vi "PulseSplitBools.vi"(1 "Pulse input":T2) -> (0 "output cluster":T1)   [LabVIEW 2017]
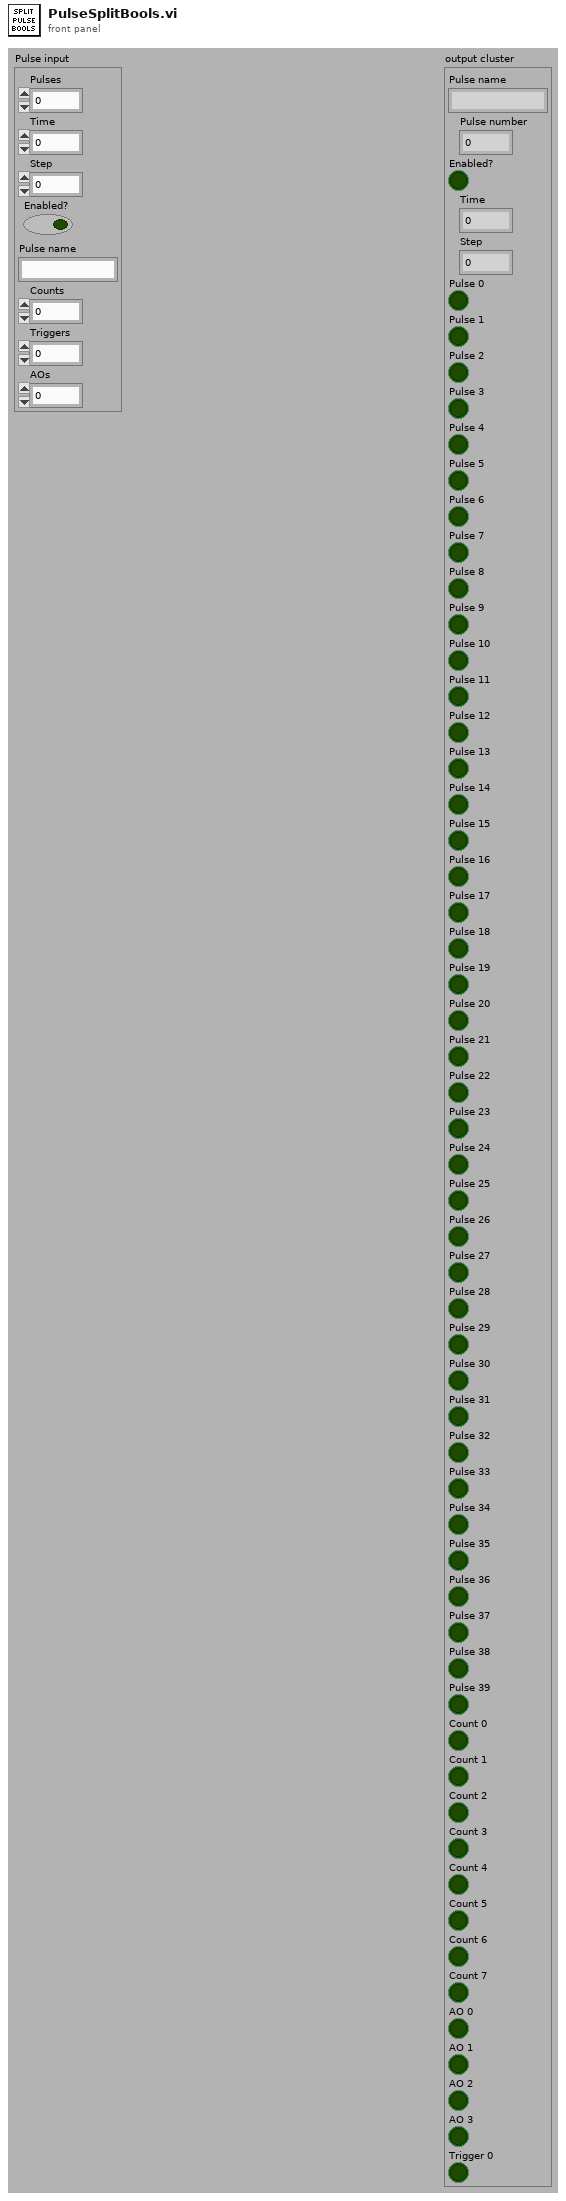
[diagram p1: front panel]
types:
  T1 = cluster{"Pulse name":string, "Pulse number":i32, "Enabled?":bool, "Time":dbl, "Step":dbl, "Pulse 0":bool, "Pulse 1":bool, "Pulse 2":bool, "Pulse 3":bool, "Pulse 4":bool, "Pulse 5":bool, "Pulse 6":bool, "Pulse 7":bool, "Pulse 8":bool, "Pulse 9":bool, "Pulse 10":bool, "Pulse 11":bool, "Pulse 12":bool, "Pulse 13":bool, "Pulse 14":bool, "Pulse 15":bool, "Pulse 16":bool, "Pulse 17":bool, "Pulse 18":bool, "Pulse 19":bool, "Pulse 20":bool, "Pulse 21":bool, "Pulse 22":bool, "Pulse 23":bool, "Pulse 24":bool, "Pulse 25":bool, "Pulse 26":bool, "Pulse 27":bool, "Pulse 28":bool, "Pulse 29":bool, "Pulse 30":bool, "Pulse 31":bool, "Pulse 32":bool, "Pulse 33":bool, "Pulse 34":bool, "Pulse 35":bool, "Pulse 36":bool, "Pulse 37":bool, "Pulse 38":bool, "Pulse 39":bool, "Count 0":bool, "Count 1":bool, "Count 2":bool, "Count 3":bool, "Count 4":bool, "Count 5":bool, "Count 6":bool, "Count 7":bool, "AO 0":bool, "AO 1":bool, "AO 2":bool, "AO 3":bool, "Trigger 0":bool}
  T2 = cluster{"Pulses":u64, "Time":dbl, "Step":dbl, "Enabled?":bool, "Pulse name":string, "Counts":u8, "Triggers":u8, "AOs":u8}
  T3 = cluster{"Boolean array[0]":bool, "Boolean array[1]":bool, "Boolean array[2]":bool, "Boolean array[3]":bool, "Boolean array[4]":bool, "Boolean array[5]":bool, "Boolean array[6]":bool, "Boolean array[7]":bool, "Boolean array[8]":bool, "Boolean array[9]":bool, "Boolean array[10]":bool, "Boolean array[11]":bool, "Boolean array[12]":bool, "Boolean array[13]":bool, "Boolean array[14]":bool, "Boolean array[15]":bool, "Boolean array[16]":bool, "Boolean array[17]":bool, "Boolean array[18]":bool, "Boolean array[19]":bool, "Boolean array[20]":bool, "Boolean array[21]":bool, "Boolean array[22]":bool, "Boolean array[23]":bool, "Boolean array[24]":bool, "Boolean array[25]":bool, "Boolean array[26]":bool, "Boolean array[27]":bool, "Boolean array[28]":bool, "Boolean array[29]":bool, "Boolean array[30]":bool, "Boolean array[31]":bool, "Boolean array[32]":bool, "Boolean array[33]":bool, "Boolean array[34]":bool, "Boolean array[35]":bool, "Boolean array[36]":bool, "Boolean array[37]":bool, "Boolean array[38]":bool, "Boolean array[39]":bool}
  T4 = cluster{"Boolean array[0]":bool, "Boolean array[1]":bool, "Boolean array[2]":bool, "Boolean array[3]":bool, "Boolean array[4]":bool, "Boolean array[5]":bool, "Boolean array[6]":bool, "Boolean array[7]":bool}
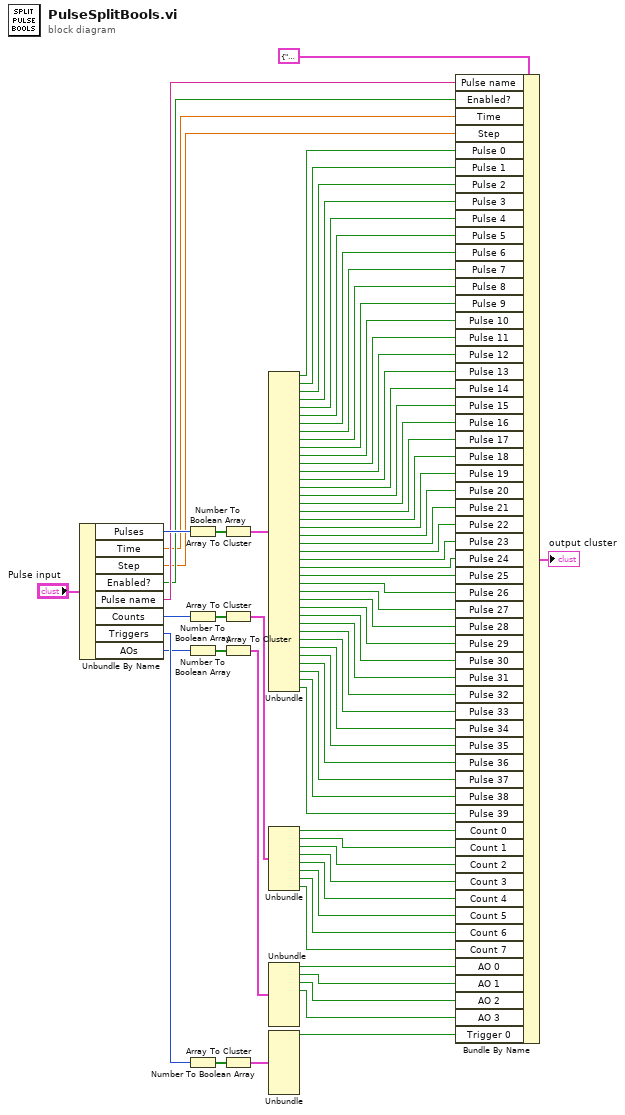
[diagram p0: block diagram]
diagram:
  n1 = Unbundle By Name("Pulse input") -> ("Pulses"=w72:u64, "Time"=w61:dbl, "Step"=w60:dbl, "Enabled?"=w62:bool, "Pulse name"=w63:string, "Counts"=w71:u8, "Triggers"=w64:u8, "AOs"=w44:u8)
  n2 = Number To Boolean Array(number=w72) -> (Boolean array=w68:bool[])
  n3 = Number To Boolean Array(number=w71) -> (Boolean array=w67:bool[])
  n4 = Number To Boolean Array(number=w44) -> (Boolean array=w45:bool[])
  n5 = Number To Boolean Array(number=w64) -> (Boolean array=w65:bool[])
  n6 = Array To Cluster(array=w68) -> (cluster=w69:T3)
  n7 = Array To Cluster(array=w67) -> (cluster=w70:T4)
  n8 = Array To Cluster(array=w45) -> (cluster=w46:T4)
  n9 = Array To Cluster(array=w65) -> (cluster=w66:T4)
  n10 = Unbundle(w69) -> ("Boolean array[0]"=w59:bool, "Boolean array[1]"=w58:bool, "Boolean array[2]"=w57:bool, "Boolean array[3]"=w56:bool, "Boolean array[4]"=w55:bool, "Boolean array[5]"=w54:bool, "Boolean array[6]"=w53:bool, "Boolean array[7]"=w52:bool, "Boolean array[8]"=w51:bool, "Boolean array[9]"=w50:bool, "Boolean array[10]"=w49:bool, "Boolean array[11]"=w48:bool, "Boolean array[12]"=w29:bool, "Boolean array[13]"=w28:bool, "Boolean array[14]"=w27:bool, "Boolean array[15]"=w26:bool, "Boolean array[16]"=w25:bool, "Boolean array[17]"=w24:bool, "Boolean array[18]"=w23:bool, "Boolean array[19]"=w22:bool, "Boolean array[20]"=w21:bool, "Boolean array[21]"=w20:bool, "Boolean array[22]"=w19:bool, "Boolean array[23]"=w18:bool, "Boolean array[24]"=w17:bool, "Boolean array[25]"=w16:bool, "Boolean array[26]"=w15:bool, "Boolean array[27]"=w14:bool, "Boolean array[28]"=w13:bool, "Boolean array[29]"=w12:bool, "Boolean array[30]"=w11:bool, "Boolean array[31]"=w10:bool, "Boolean array[32]"=w9:bool, "Boolean array[33]"=w8:bool, "Boolean array[34]"=w7:bool, "Boolean array[35]"=w6:bool, "Boolean array[36]"=w5:bool, "Boolean array[37]"=w4:bool, "Boolean array[38]"=w3:bool, "Boolean array[39]"=w2:bool)
  n11 = Unbundle(w70) -> ("Boolean array[0]"=w42:bool, "Boolean array[1]"=w41:bool, "Boolean array[2]"=w40:bool, "Boolean array[3]"=w39:bool, "Boolean array[4]"=w38:bool, "Boolean array[5]"=w37:bool, "Boolean array[6]"=w36:bool, "Boolean array[7]"=w34:bool)
  n12 = Unbundle(w46) -> ("Boolean array[0]"=w35:bool, "Boolean array[1]"=w33:bool, "Boolean array[2]"=w32:bool, "Boolean array[3]"=w31:bool)  [unwired: 4 out]
  n13 = Unbundle(w66) -> ("Boolean array[0]"=w30:bool)  [unwired: 7 out]
  n14 = Bundle By Name(cluster=T1 {"Pulse name"="", "Pulse number"=0, "Enabled?"=FALSE, "Time"=0.0, "Step"=0.0, "Pulse 0"=FALSE, "Pulse 1"=FALSE, "Pulse 2"=FALSE, "Pulse 3"=FALSE, "Pulse 4"=FALSE, "Pulse 5"=FALSE, "Pulse 6"=FALSE, "Pulse 7"=FALSE, "Pulse 8"=FALSE, "Pulse 9"=FALSE, "Pulse 10"=FALSE, "Pulse 11"=FALSE, "Pulse 12"=FALSE, "Pulse 13"=FALSE, "Pulse 14"=FALSE, "Pulse 15"=FALSE, "Pulse 16"=FALSE, "Pulse 17"=FALSE, "Pulse 18"=FALSE, "Pulse 19"=FALSE, "Pulse 20"=FALSE, "Pulse 21"=FALSE, "Pulse 22"=FALSE, "Pulse 23"=FALSE, "Pulse 24"=FALSE, "Pulse 25"=FALSE, "Pulse 26"=FALSE, "Pulse 27"=FALSE, "Pulse 28"=FALSE, "Pulse 29"=FALSE, "Pulse 30"=FALSE, "Pulse 31"=FALSE, "Pulse 32"=FALSE, "Pulse 33"=FALSE, "Pulse 34"=FALSE, "Pulse 35"=FALSE, "Pulse 36"=FALSE, "Pulse 37"=FALSE, "Pulse 38"=FALSE, "Pulse 39"=FALSE, "Count 0"=FALSE, "Count 1"=FALSE, "Count 2"=FALSE, "Count 3"=FALSE, "Count 4"=FALSE, "Count 5"=FALSE, "Count 6"=FALSE, "Count 7"=FALSE, "AO 0"=FALSE, "AO 1"=FALSE, "AO 2"=FALSE, "AO 3"=FALSE, "Trigger 0"=FALSE} ("Raw pulse"), "Pulse name"=w63, "Enabled?"=w62, "Time"=w61, "Step"=w60, "Pulse 0"=w59, "Pulse 1"=w58, "Pulse 2"=w57, "Pulse 3"=w56, "Pulse 4"=w55, "Pulse 5"=w54, "Pulse 6"=w53, "Pulse 7"=w52, "Pulse 8"=w51, "Pulse 9"=w50, "Pulse 10"=w49, "Pulse 11"=w48, "Pulse 12"=w29, "Pulse 13"=w28, "Pulse 14"=w27, "Pulse 15"=w26, "Pulse 16"=w25, "Pulse 17"=w24, "Pulse 18"=w23, "Pulse 19"=w22, "Pulse 20"=w21, "Pulse 21"=w20, "Pulse 22"=w19, "Pulse 23"=w18, "Pulse 24"=w17, "Pulse 25"=w16, "Pulse 26"=w15, "Pulse 27"=w14, "Pulse 28"=w13, "Pulse 29"=w12, "Pulse 30"=w11, "Pulse 31"=w10, "Pulse 32"=w9, "Pulse 33"=w8, "Pulse 34"=w7, "Pulse 35"=w6, "Pulse 36"=w5, "Pulse 37"=w4, "Pulse 38"=w3, "Pulse 39"=w2, "Count 0"=w42, "Count 1"=w41, "Count 2"=w40, "Count 3"=w39, "Count 4"=w38, "Count 5"=w37, "Count 6"=w36, "Count 7"=w34, "AO 0"=w35, "AO 1"=w33, "AO 2"=w32, "AO 3"=w31, "Trigger 0"=w30) -> (→"output cluster":T1)
